vi "Append Fail Result.vi"(7 "Description":string, 8 "error in (no error)":errorcluster, 9 "Message":string, 10 "Result Type":T1, 11 "LUnit Test Case In":refnum<class "LUnit Test Case V2.lvclass">) -> (0 "error out":errorcluster, 3 "LUnit Test Case Out":refnum<class "LUnit Test Case V2.lvclass">)   [LabVIEW 2020, in "LUnit Test Case V2.lvclass"]
doc: "Generates a fail result for the calling test method. A description and message may be provided."
uses:
  LUnit Test Case V2.lvclass
  Result/Type.ctl
  Result/Result.ctl
  Result/Status.ctl
  LUnit Test Case V2.lvclass/LUnit Test Case V2.ctl
  Result/Result.lvlib
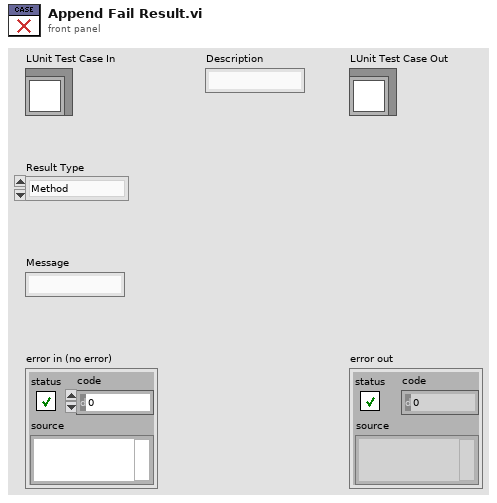
[diagram p1: front panel]
types:
  T1 = typedef "Result.lvlib/Type.ctl" = enum16{"Method", "Case", "Suite", "Pass", "Fail", "Skip", "Pass if", "Fail if", "Pass if Error", "Fail if Error", "Pass if Equal", "Fail if Equal"}
  T2 = typedef "Result.lvlib/Result.ctl" = cluster{"Name":string, "Message":string, "Description":string, "Status":T3, "Result Type":T1, "Execution Time":dbl}
  T3 = typedef "Result.lvlib/Status.ctl" = enum16{"", "Passed", "Failed", "Error", "Skipped", "Setup Error", "Broken", "Teardown Error"}
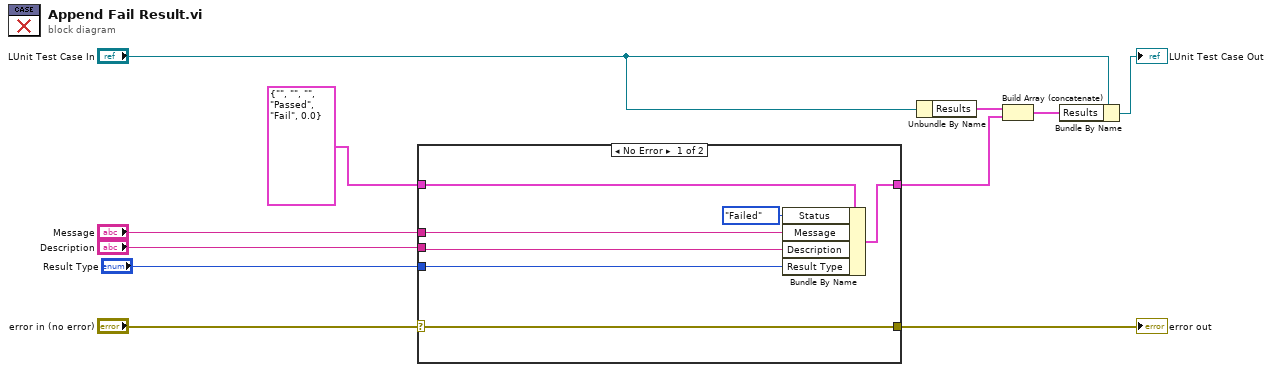
[diagram p0: block diagram]
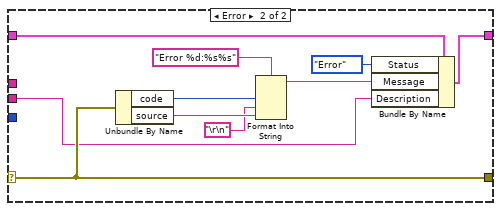
[diagram p2: hidden frame]
diagram:
  n1 = case shown="No Error" "error in (no error)" {
    selector: "error in (no error)" -> [w16 w24]
    tunnel: T2 {"Name"="", "Message"="", "Description"="", "Status"=enum."Passed", "Result Type"=enum."Fail", "Execution Time"=0.0} ("Temporary Assertion Result") -> [w18 w21]
    tunnel: [w17 w22] -> w4
    tunnel: [w16 w24] -> w8
    tunnel: "Message" -> [w15 _]
    tunnel: "Description" -> [w14 w20]
    tunnel: "Result Type" -> [w12 _]
    frame No Error {
      n2 = Bundle By Name(cluster=w18, "Status"=Status."Failed", "Message"=w15, "Description"=w14, "Result Type"=w12) -> (w17:T2)
    }
    frame Error {
      n3 = Unbundle By Name(w24) -> ("code"=w28:i32, "source"=w26:string)
      n4 = Format Into String(format string="Error %d:%s%s", w28, "\r\n", w26) -> (resulting string=w27:string)  [unwired: 2 in, 1 out]
      n5 = Bundle By Name(cluster=w21, "Status"=Status."Error", "Message"=w27, "Description"=w20) -> (w22:T2)
    }
  }
  "error out" <- w8
  n6 = Unbundle By Name("LUnit Test Case In") -> ("Results"=w2:T2[])
  n7 = Build Array (concatenate)(w2, w4) -> (w1:T2[])
  n8 = Bundle By Name(cluster="LUnit Test Case In", "Results"=w1) -> (→"LUnit Test Case Out":refnum<class "LUnit Test Case V2.lvclass">)
